vi "ULx Write (Counter Frequency 1Chan 1Samp).vi"(0 "task in":refnum<k24>, 1 "auto start":bool=TRUE, 5 "frequency":dbl=1.0 format="%_6g", 7 "duty cycle":dbl=0.5 format="%_6g", 9 "timeout":dbl=10.0 format="%_4g", 11 "error in":errorcluster) -> (4 "task out":refnum<k24>, 10 "number of samples written per channel":u32, 15 "error out":errorcluster)   [LabVIEW 2020]
doc: "Writes a new pulse frequency and duty cycle to a counter output task that contains a single channel."
uses:
  C:/Users/William/Documents/LV 2020 builds/LeaktestDAQ/Source-v33/ULx_LV.dll
  ULx_LV.dll
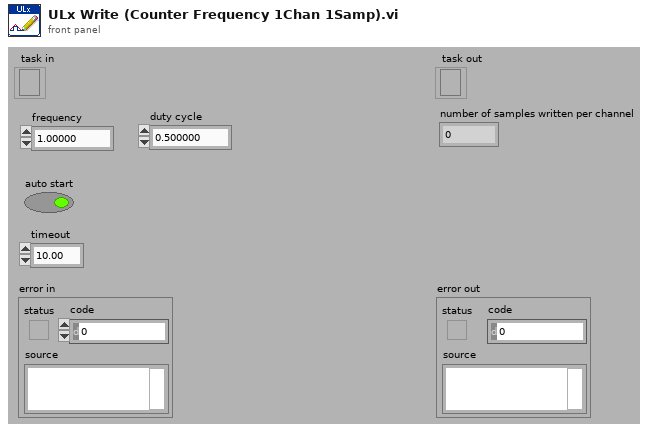
[diagram p1: front panel]
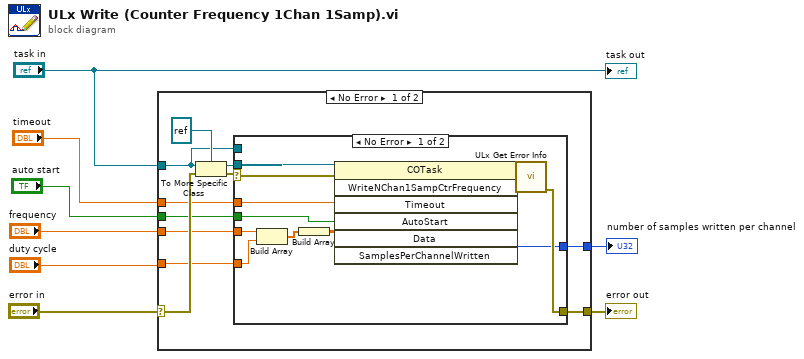
[diagram p0: block diagram]
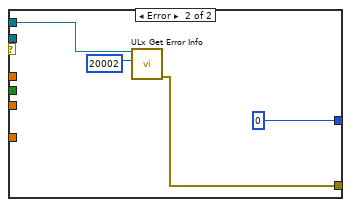
[diagram p2: hidden frame]
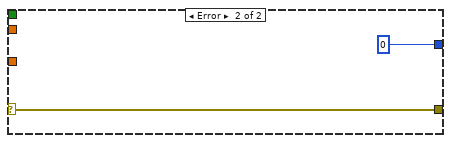
[diagram p3: hidden frame]
diagram:
  n1 = case shown="No Error" "error in" {
    selector: "error in" -> [w19 w38]
    tunnel: "task in" -> [w13 _]
    tunnel: "timeout" -> [w15 _]
    tunnel: [w14 w38] -> w6
    tunnel: "auto start" -> [w12 _]
    tunnel: [w11 0 ("SamplesPerChannelWritten")] -> w3
    tunnel: "duty cycle" -> [w9 _]
    tunnel: "frequency" -> [w10 _]
    frame No Error {
      n2 = To More Specific Class(target class=refnum<k24> refnum, reference=w13, error in=w19) -> (specific class reference=w16:refnum<k24>, error out=w17:errorcluster)
      n3 = case shown="No Error" w17 {
        selector: w17 -> [w31 _]
        tunnel: w16 -> [w32 _]
        tunnel: w15 -> [w25 _]
        tunnel: [w28 w35] -> w14
        tunnel: w13 -> [_ w34]
        tunnel: w12 -> [w24 _]
        tunnel: [w26 0 ("SamplesPerChannelWritten")] -> w11
        tunnel: w10 -> [w22 _]
        tunnel: w9 -> [w23 _]
        frame No Error {
          n4 = Build Array(w22, w23) -> (w21:dbl[])
          n5 = Build Array(w21) -> (w20:dbl[][])
          n6 = invoke class="COTask" method="WriteNChan1SampCtrFrequency"(reference=w32, error in=w31, "Timeout"=w25, "AutoStart"=w24, "Data"=w20) -> (reference out=w29:refnum<k24>, error out=w30:errorcluster, "WriteNChan1SampCtrFrequency"=w27:i32, "SamplesPerChannelWritten"=w26:u32)  [unwired: 2 in, 3 out]
          n7 = call "ULx Get Error Info.vi"("error in"=w30, "ErrorCode"=w27, "task in"=w29) -> ("error out"=w28:errorcluster)  [unwired: 8 in]
        }
        frame Error {
          n8 = call "ULx Get Error Info.vi"("ErrorCode"=20002, "task in"=w34) -> ("error out"=w35:errorcluster)  [unwired: 9 in]
        }
      }
    }
    frame Error {
    }
  }
  "error out" <- w6
  "number of samples written per channel" <- w3
  "task out" <- "task in"
